vi "mupExpr sglExpr sglVar example.vi"() -> ()   [LabVIEW 2015]
uses:
  mupExpr/mupExpr.lvclass
  mupExpr/mupExpr.lvclass/mupExpr.ctl
  mupExpr/Eval_SglVar_SglRes.vi
  mupLib/mupEval.vi
  mupLib/mupSetVarValue.vi
  mupLib/mupCheckError.vi
  mupLib/mupLibPath.vi
  <vilib>/Utility/error.llb/Error Cluster From Error Code.vi
panel:
  out "Result":dbl
  in  "Variable Value":dbl=1.0 format="%#_13g"
  out "error out":errorcluster
  in  "Expression":string="1*x^2+2*x+3"
  # "This example demonstrates the basic usage of mupExpr.\nIt will evaluate the input expression assuming a single variable.\nIf the expression contains more than one variable, the result will be NaN.\n\n- Enter an expression composed up to one variable\n- Enter the value of the variable\n- Hit run to evaluate the expression"
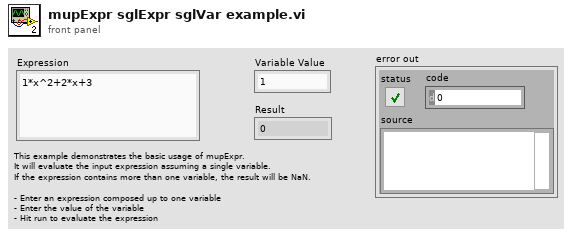
[diagram p1: front panel]
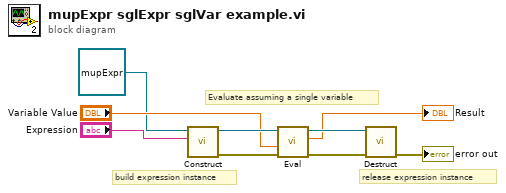
[diagram p0: block diagram]
diagram:
  # "release expression instance"
  # "build expression instance"
  # "Evaluate assuming a single variable"
  n1 = call-dynamic "Construct.vi"("Expression"="Expression", "muExpr in"=refnum<class "mupExpr.lvclass"> refnum) -> ("error out"=w5:errorcluster, "mupExpr out"=w4:refnum<class "mupExpr.lvclass">)  [unwired: 6 in, 2 out]
  n2 = call-poly "Eval.vi"("error in (no error)"=w5, "varValue"="Variable Value", "muExpr in"=w4) -> ("error out"=w7:errorcluster, "Result"=→"Result":dbl, "muExpr out"=w8:refnum<class "mupExpr.lvclass">)  [unwired: 6 in]
  n3 = call-dynamic "Destruct.vi"("error in (no error)"=w7, "muExpr in"=w8) -> ("error out"=→"error out":errorcluster)  [unwired: 9 in]
